vi "Main.vi"(11 "Module Admin":refnum<class "Delacor_lib_QMH_Module Admin.lvclass">) -> ()   [LabVIEW 2024, in "ProductControl.lvlib"]
doc: "This template is based off of the Queued Message Handler design pattern and the Queued Message Handler project template that ships with LabVIEW.\n\nThe main difference is that the queue is private to this module and communication between modules is performed via Broadcast and Request events.\n\nRequest events are wrapped in public API methods and are handled in the Event Handling Loop (EHL) of this VI. Any module can register for Broadcast events sent by this module. The EHL generates messages based on user interface actions.\n\nThe Message Handling Loop (MHL) processes messages generated by the EHL, or by other messages. The messages are string values, so new messages can be added easily to the Message Cases case structure in the MHL. Each message cluster can also provide an optional value for Message Data, which is a variant that can be converted to whatever message-specific data is required.\n_____\nBased on DQMH Dev Tools: Project Template 7.1.0.1503."
uses:
  ProductControl.lvlib
  <vilib>/Delacor/Delacor QMH/Libraries/Module Admin_class/Delacor_lib_QMH_Module Admin.lvclass
  Module Data--cluster.ctl
  <vilib>/Utility/miscctls.llb/LVFontTypeDef.ctl
  Stop Argument--cluster.ctl
  <vilib>/Delacor/Delacor QMH/Libraries/Message Queue_class/Delacor_lib_QMH_Message Queue.lvclass/Delacor_lib_QMH_Message Queue.ctl
  <vilib>/Delacor/Delacor QMH/Libraries/Module Admin_class/Delacor_lib_QMH_Module Admin.lvclass/Delacor_lib_QMH_Module Admin.ctl
  Draw FP in Subpanel Argument--cluster.ctl
  Remove From Subpanel Argument--cluster.ctl
  <vilib>/Delacor/Delacor QMH/Libraries/Message Queue_class/Delacor_lib_QMH_Enqueue Message (Single).vi
  <vilib>/Delacor/Delacor QMH/Libraries/Module Admin_class/Delacor_lib_QMH_Get External Launch.vi
  <vilib>/Delacor/Delacor QMH/Libraries/Message Queue_class/Delacor_lib_QMH_Message Queue.lvclass
  <vilib>/PantherLAB/Message Module/Libraries/Message/PantherLAB_lib_Message.lvlib
panel:
  in  "Productos":i32(listbox)
  out "error out":errorcluster
  out "Status":string
  in  "Comprar":bool
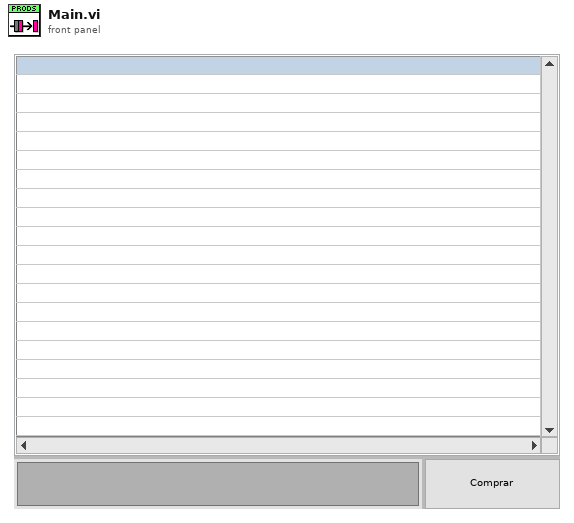
[diagram p1: front panel]
types:
  T1 = typedef "ProductControl.lvlib/Request Events--cluster.ctl" = cluster{"Stop Module":refnum<user-event>, "Show Panel":refnum<user-event>, "Hide Panel":refnum<user-event>, "Get Module Execution Status":refnum<user-event>, "Show Diagram":refnum<user-event>, "Draw FP in Subpanel":refnum<user-event>, "Remove From Subpanel":refnum<user-event>}
  T2 = typedef "PantherLAB_lib_Message.lvlib/Broadcast Events--cluster.ctl" = cluster{"Module Did Init":refnum<user-event>, "Status Updated":refnum<user-event>, "Error Reported":refnum<user-event>, "Module Did Stop":refnum<user-event>, "Update Module Execution Status":refnum<user-event>}
  T3 = typedef "ProductControl.lvlib/Module Data--cluster.ctl" = cluster{"Status":string, "Sub Panel":refnum<vi>}
  T4 = typedef "LVFontTypeDef.ctl" = cluster{"Font Name":string, "Size":u16, "Bold":bool, "Italic":bool, "Underline":bool, "Strikeout":bool, "Color":u32}
  T5 = enum32{"invalid lock state", "Not Locked", "Locked (No Password)", "Password-protected"}
  T6 = typedef "ProductControl.lvlib/Stop Argument--cluster.ctl" = cluster{"Origin":string, "Exit via Stop Module Req?":bool, "Wait for Module to stop?":bool}
  T7 = typedef "ProductControl.lvlib/Draw FP in Subpanel Argument--cluster.ctl" = cluster{"Sub Panel":refnum<vi>}
  T8 = typedef "ProductControl.lvlib/Remove From Subpanel Argument--cluster.ctl" = cluster{"Boolean":bool}
  T9 = enum32{"Invalid", "Standard", "Closed", "Hidden", "Minimized", "Maximized"}
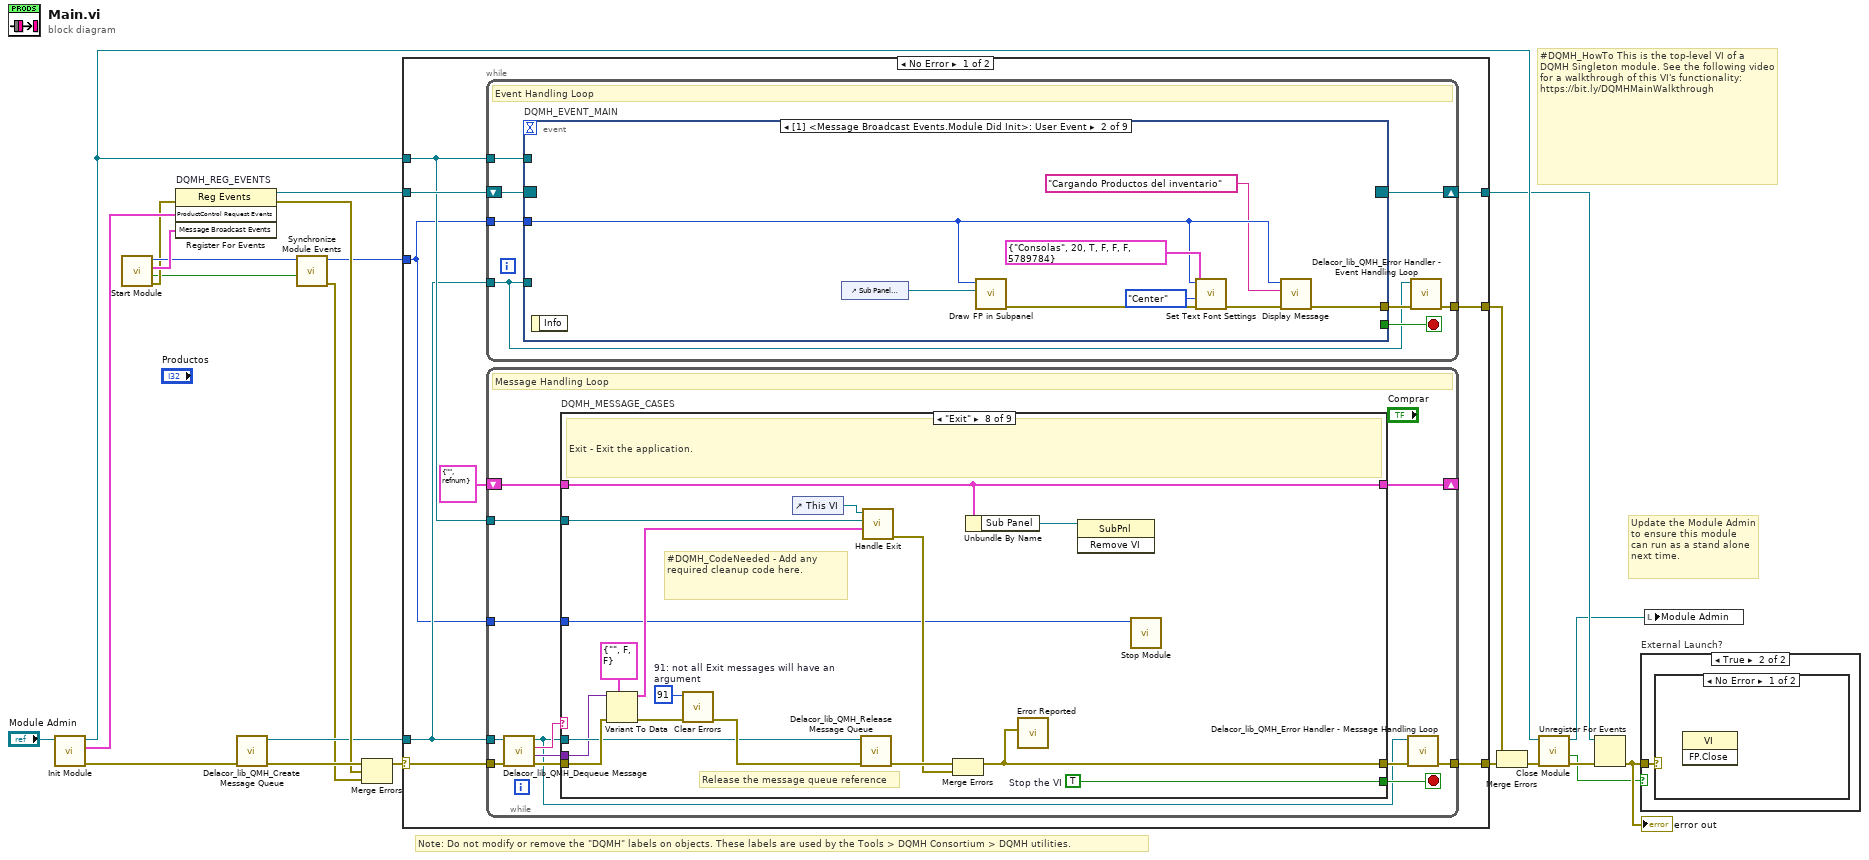
[diagram p0: block diagram]
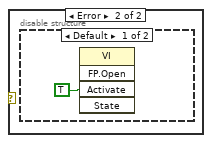
[diagram p3: hidden frame]
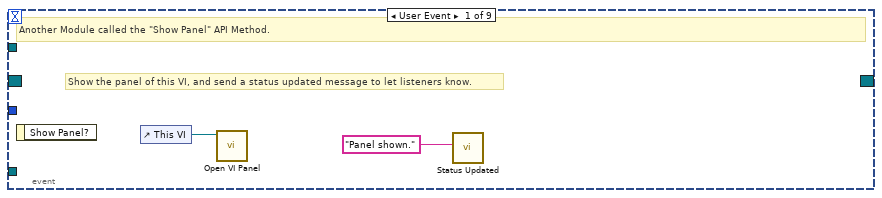
[diagram p5: hidden frame]
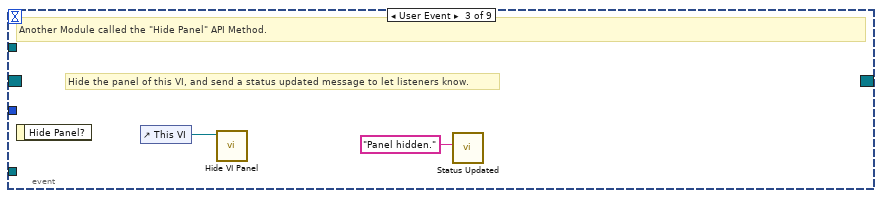
[diagram p6: hidden frame]
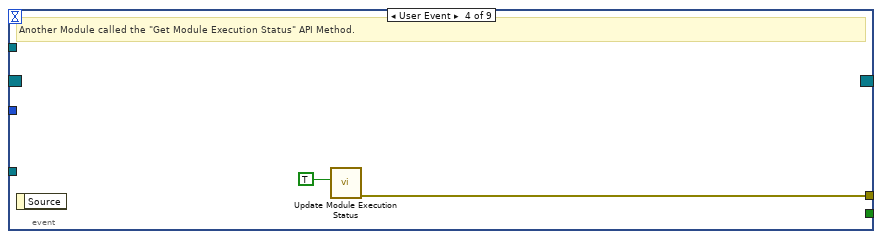
[diagram p7: hidden frame]
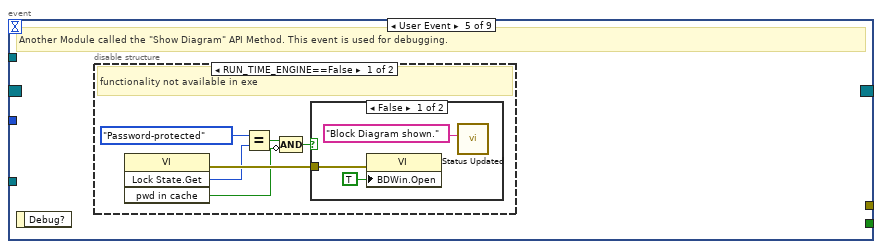
[diagram p8: hidden frame]
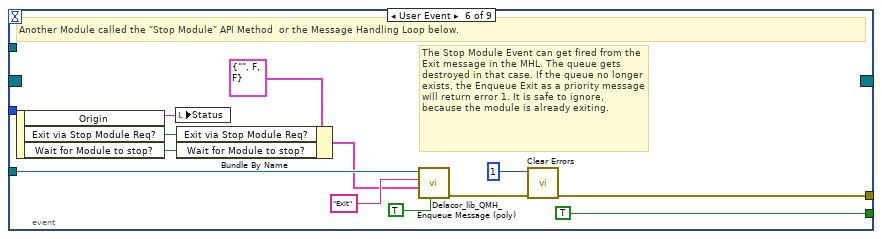
[diagram p11: hidden frame]
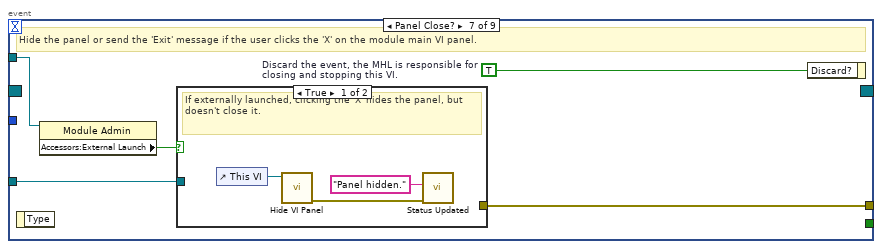
[diagram p12: hidden frame]
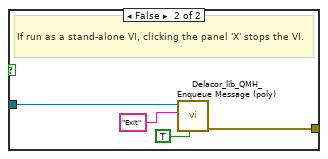
[diagram p13: hidden frame]
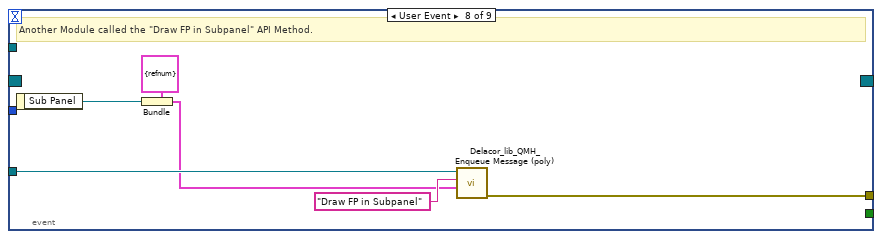
[diagram p14: hidden frame]
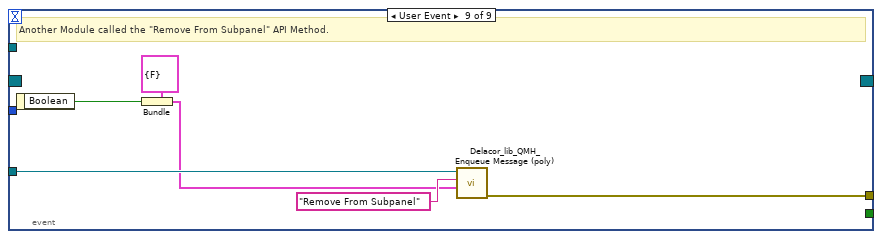
[diagram p15: hidden frame]
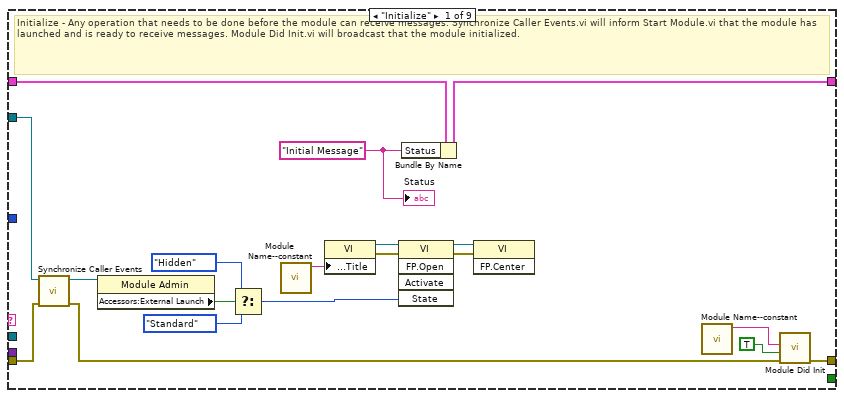
[diagram p16: hidden frame]
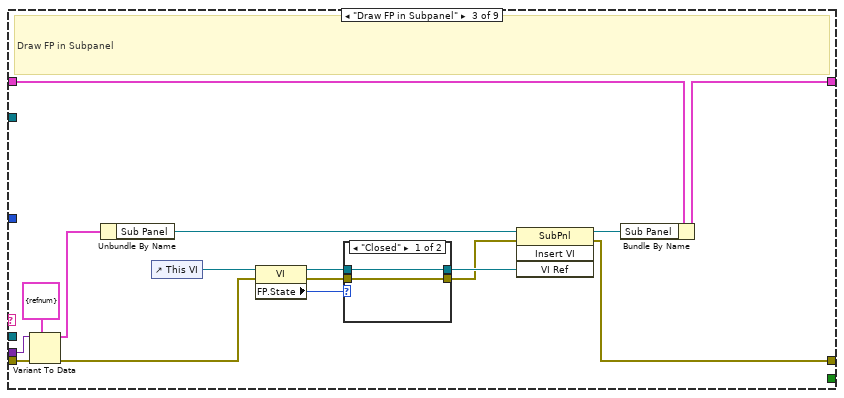
[diagram p18: hidden frame]
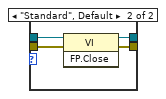
[diagram p19: hidden frame]
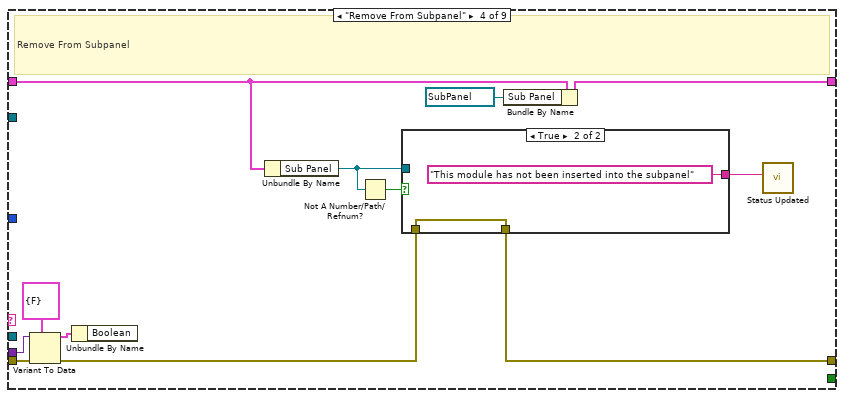
[diagram p20: hidden frame]
diagram:
  # "#DQMH_HowTo This is the top-level VI of a DQMH Singleton module. See the following video for a walkthrough of this VI's functionality: https://bit.ly/DQMHMainWalkthrough"
  # "Note: Do not modify or remove the \"DQMH\" labels on objects. These labels are used by the Tools > DQMH Consortium > DQMH utilities."
  # "Update the Module Admin to ensure this module can run as a stand alone next time."
  n1 = call "Init Module.vi"("Singleton Module Admin in"="Module Admin") -> ("error out"=w22:errorcluster, "ProductControl Request Events"=w11:T1, "Singleton Module Admin out"=w14:refnum<class "Delacor_lib_QMH_Module Admin.lvclass">)  [unwired: 8 in]
  n2 = call <vilib>:"Start Module.vi"() -> ("error out"=w4:errorcluster, "Wait for Event Sync?"=w3:bool, "Message Broadcast Events"=w6:T2, "Module ID"=w5:i32)  [unwired: 7 in, 1 out]
  n3 = register-events "DQMH_REG_EVENTS"(error in=w4, w11, w6) -> (reference out=w12:refnum<event-registration>, error out=w15:errorcluster)  [unwired: 1 in]
  n4 = call <vilib>:"Delacor_lib_QMH_Create Message Queue.vi"("error in"=w22) -> ("error out"=w17:errorcluster, "Message Queue"=w10:refnum<class "Delacor_lib_QMH_Message Queue.lvclass">)  [unwired: 9 in]
  n5 = call <vilib>:"Synchronize Module Events.vi"("Wait for Event Sync?"=w3, "Module ID in"=w5) -> ("error out"=w1:errorcluster, "Module ID out"=w2:i32)  [unwired: 8 in]
  n6 = Merge Errors(w17, w15, w1) -> (w16:errorcluster)
  n7 = case shown="No Error" w16 {
    selector: w16 -> [w30 w231]
    tunnel: [w32 w230] -> w23
    tunnel: [w29 w229] -> w13
    tunnel: w12 -> [w27 w229]
    tunnel: w10 -> [w25 w225]
    tunnel: [w31 _] -> w20
    tunnel: w14 -> [w26 w226]
    tunnel: w2 -> [w24 w224]
    frame No Error {
      n8 = while {
        tunnel: w25 -> [w34]
        shift-right: [w37] -> w29
        shift-left: w27 -> [w38]
        tunnel: [w39] -> w31
        tunnel: w26 -> [w35]
        tunnel: w24 -> [w33]
        stop <- w36 stop-if-true
        # "Event Handling Loop"
        n9 = event "DQMH_EVENT_MAIN" shown="[1] <Message Broadcast Events.Module Did Init>: User Event" {
          selector: w38 -> [_ _ _ _ _ _ _ _ _]
          dyn-events: [_ _ _ _ _ _ _ _ _] -> w37
          timeout: _ -> [_ _ _ _ _ _ _ _ _]
          tunnel: [_ _ _ _ _ TRUE ("Discard?") _ _ _] -> w36
          tunnel: w34 -> [_ _ _ _ _ w71 w78 w93 w99]
          tunnel: [_ w45 _ w54 _ w74 w80 w88 w94] -> w40
          tunnel: w35 -> [_ _ _ _ _ _ w77 _ _]
          tunnel: w33 -> [_ w44 _ _ _ _ _ _ _]
          event User Event {
            # "Show the panel of this VI, and send a status updated message to let listeners know."
            # "Another Module called the \"Show Panel\" API Method."
            n10 = event-data() -> ()  [unwired: 1 in, 1 out]
            n11 = control-ref of="This VI"() -> (w42:refnum<vi>)
            n12 = call "Open VI Panel.vi"("VI"=w42) -> ()  [unwired: 10 in, 1 out]
            n13 = call "Status Updated.vi"("Status"="Panel shown." ("format string")) -> ()  [unwired: 10 in, 1 out]
          }
          event User Event {
            n14 = event-data() -> ()  [unwired: 1 in, 1 out]
            n15 = control-ref of="Sub Panel Mensajes"() -> (w50:refnum<vi>)
            n16 = call <vilib>:"Draw FP in Subpanel.vi"("Sub Panel"=w50, "Module ID"=w44) -> ("error out"=w49:errorcluster)  [unwired: 9 in]
            n17 = call <vilib>:"Set Text Font Settings.vi"("error in"=w49, "Text.Justification"=enum16{"Left", "Center", "Right"}."Center", "Font"=T4 {"Font Name"="Consolas", "Size"=20, "Bold"=TRUE, "Italic"=FALSE, "Underline"=FALSE, "Strikeout"=FALSE, "Color"=5789784}, "Module ID"=w44) -> ("error out"=w46:errorcluster)  [unwired: 7 in]
            n18 = call <vilib>:"Display Message.vi"("error in"=w46, "Message"="Cargando Productos del inventario", "Module ID"=w44) -> ("error out"=w45:errorcluster)  [unwired: 8 in]
          }
          event User Event {
            # "Hide the panel of this VI, and send a status updated message to let listeners know."
            # "Another Module called the \"Hide Panel\" API Method."
            n19 = event-data() -> ()  [unwired: 1 in, 1 out]
            n20 = control-ref of="This VI"() -> (w52:refnum<vi>)
            n21 = call "Hide VI Panel.vi"("VI"=w52) -> ()  [unwired: 10 in, 1 out]
            n22 = call "Status Updated.vi"("Status"="Panel hidden." ("format string")) -> ()  [unwired: 10 in, 1 out]
          }
          event User Event {
            # "Another Module called the \"Get Module Execution Status\" API Method."
            n23 = event-data() -> ()  [unwired: 1 in, 1 out]
            n24 = call "Update Module Execution Status.vi"("Running?"=TRUE) -> ("error out"=w54:errorcluster)  [unwired: 10 in]
          }
          event User Event {
            # "Another Module called the \"Show Diagram\" API Method. This event is used for debugging."
            n25 = event-data() -> ()  [unwired: 1 in, 1 out]
            n26 = disable-structure shown="RUN_TIME_ENGINE==False" {
              frame condition #0 (active) {
                # "functionality not available in exe"
                n27 = invoke on="Invoke Node" class="VI" method="Lock State.Get"() -> (error out=w60:errorcluster, "Get Lock State"=w59:T5, "pwd in cache"=w56:bool)  [unwired: 4 in, 1 out]
                n28 = Equal?(x=T5."Password-protected", y=w59) -> (x = y?=w57:bool)
                n29 = Compound Arithmetic op=AND(w57, invert w56) -> (w55:bool)
                n30 = case shown="False" w55 {
                  tunnel: w60 -> [w63 _]
                  frame False {
                    n31 = property on="Property Node" class="VI"(error in=w63, "BDWin.Open"=TRUE ("Block Diagram Window:Open")) -> ()  [unwired: 1 in, 2 out]
                    n32 = call "Status Updated.vi"("Status"="Block Diagram shown." ("format string")) -> ()  [unwired: 10 in, 1 out]
                  }
                  frame True {
                    # "Password-protected VI, and the password is not in the cache. Do not show the diagram."
                  }
                }
              }
              frame condition #1 {
              }
            }
          }
          event User Event {
            # "The Stop Module Event can get fired from the Exit message in the MHL. The queue gets destroyed in that case. If the queue no longer exists, the Enqueue Exit as a priority message will return error 1. It is safe to ignore, because the module is already exiting."
            # "Another Module called the \"Stop Module\" API Method  or the Message Handling Loop below."
            n33 = event-data() -> ("Origin"=w70:string, "Exit via Stop Module Req?"=w66:bool, "Wait for Module to stop?"=w65:bool)  [unwired: 1 in]
            n34 = local write "Status"(w70) -> ()
            n35 = Bundle By Name(cluster=T6 {"Origin"="", "Exit via Stop Module Req?"=FALSE, "Wait for Module to stop?"=FALSE} ("Stop Argument"), "Exit via Stop Module Req?"=w66, "Wait for Module to stop?"=w65) -> (w64:T6)
            n36 = call-poly <vilib>:"Delacor_lib_QMH_Enqueue Message (poly).vi"("Priority Message? (F)"=TRUE, "Message Data"=w64, "Message"="Exit", "Message Queue in"=w71) -> ("error out"=w75:errorcluster)  [unwired: 6 in, 1 out]
            n37 = call <vilib>:"Clear Errors.vi"("error in (no error)"=w75, "specific error code to clear (0: all)"=1) -> ("error out"=w74:errorcluster)  [unwired: 4 in, 1 out]
          }
          event Panel Close? {
            w79 = TRUE  # Discard the event, the MHL is responsible for closing and stopping this VI.
            # "Hide the panel or send the 'Exit' message if the user clicks the 'X' on the module main VI panel."
            n38 = event-data() -> ()  [unwired: 1 in, 1 out]
            n39 = property on="Property Node" class="Module Admin"(reference=w77) -> ("Accessors:External Launch"=w76:bool)  [unwired: 1 in, 2 out]
            n40 = case shown="True" w76 {
              tunnel: w78 -> [_ w86]
              tunnel: [_ w87] -> w80
              frame True {
                # "If externally launched, clicking the 'X' hides the panel, but doesn't close it."
                n41 = control-ref of="This VI"() -> (w83:refnum<vi>)
                n42 = call "Hide VI Panel.vi"("VI"=w83) -> ("error out"=w81:errorcluster)  [unwired: 10 in]
                n43 = call "Status Updated.vi"("error in"=w81, "Status"="Panel hidden." ("format string")) -> ()  [unwired: 9 in, 1 out]
              }
              frame False {
                # "If run as a stand-alone VI, clicking the panel 'X' stops the VI."
                n44 = call-poly <vilib>:"Delacor_lib_QMH_Enqueue Message (poly).vi"("Priority Message? (F)"=TRUE, "Message"="Exit", "Message Queue in"=w86) -> ("error out"=w87:errorcluster)  [unwired: 7 in, 1 out]
              }
            }
            n45 = event-data ("Event Filter Node")("Discard?"=w79) -> ()  [unwired: 1 in, 1 out]
          }
          event User Event {
            # "Another Module called the \"Draw FP in Subpanel\" API Method."
            n46 = event-data() -> ("Sub Panel"=w89:refnum<vi>)  [unwired: 1 in]
            n47 = Bundle(cluster=T7 {"Sub Panel"=refnum} ("Draw FP in Subpanel Argument"), "Sub Panel"=w89) -> (w90:T7)
            n48 = call-poly <vilib>:"Delacor_lib_QMH_Enqueue Message (poly).vi"("Message Data"=w90, "Message"="Draw FP in Subpanel", "Message Queue in"=w93) -> ("error out"=w88:errorcluster)  [unwired: 7 in, 1 out]
          }
          event User Event {
            # "Another Module called the \"Remove From Subpanel\" API Method."
            n49 = event-data() -> ("Boolean"=w95:bool)  [unwired: 1 in]
            n50 = Bundle(cluster=T8 {"Boolean"=FALSE} ("Remove From Subpanel Argument"), "Boolean"=w95) -> (w96:T8)
            n51 = call-poly <vilib>:"Delacor_lib_QMH_Enqueue Message (poly).vi"("Message Data"=w96, "Message"="Remove From Subpanel", "Message Queue in"=w99) -> ("error out"=w94:errorcluster)  [unwired: 7 in, 1 out]
          }
        }
        n52 = call-dynamic "Delacor_lib_QMH_Error Handler - Event Handling Loop.vi"("error in"=w40, "Message Queue in"=w34) -> ("dup error in"=w39:errorcluster)  [unwired: 8 in, 1 out]
      }
      n53 = while {
        tunnel: w25 -> [w101]
        shift-right: [w109] -> _
        shift-left: T3 {"Status"="", "Sub Panel"=refnum} ("Data Cluster") -> [w110]
        tunnel: w30 -> [w112]
        tunnel: [w104] -> w32
        tunnel: w26 -> [w105]
        tunnel: w24 -> [w100]
        stop <- w108 stop-if-true
        # "Message Handling Loop"
        n54 = call-dynamic "Delacor_lib_QMH_Dequeue Message.vi"("error in"=w112, "Message Queue in"=w101) -> ("error out"=w111:errorcluster, "Message Data"=w106:variant, "Message"=w107:string, "Message Queue out"=w102:refnum<class "Delacor_lib_QMH_Message Queue.lvclass">)  [unwired: 6 in]
        n55 = case "DQMH_MESSAGE_CASES" shown="\"Exit\"" w107 {
          selector: w107 -> [_ _ _ _ _ _ _ _ w218]
          tunnel: w102 -> [_ _ _ _ _ _ w182 w206 _]
          tunnel: w111 -> [w129 w133 w149 w167 w176 w178 w189 w212 w221]
          tunnel: [w127 w133 w141 w161 w175 w178 w185 w207 w222] -> w103
          tunnel: w110 -> [w118 w132 w148 w163 w174 w177 w184 w198 w219]
          tunnel: [w117 w132 w144 w158 w174 w177 w184 w198 w219] -> w109
          tunnel: [_ _ _ _ _ _ _ w205 _] -> w108
          tunnel: w106 -> [_ _ w147 w166 _ _ w183 w204 _]
          tunnel: w105 -> [w119 _ _ _ _ _ w181 w199 _]
          tunnel: w100 -> [_ _ _ _ _ _ _ w196 _]
          frame "Initialize" {
            w113 = "Initial Message" ("Initial Message")
            # "Initialize - Any operation that needs to be done before the module can receive messages. Synchronize Caller Events.vi will inform Start Module.vi that the module has launched and is ready to receive messages. Module Did Init.vi will broadcast that the module initialized."
            n56 = call "Synchronize Caller Events.vi"("error in"=w129, "Singleton Module Admin in"=w119) -> ("error out"=w128:errorcluster, "Singleton Module Admin out"=w114:refnum<class "Delacor_lib_QMH_Module Admin.lvclass">)  [unwired: 8 in]
            n57 = property on="Property Node" class="Module Admin"(reference=w114) -> ("Accessors:External Launch"=w123:bool)  [unwired: 1 in, 2 out]
            n58 = Select(t=T9."Hidden" ("State"), s=w123, f=T9."Standard" ("State")) -> (s? t:f=w120:T9)
            n59 = call "Module Name--constant.vi"() -> ("Module Name"=w126:string)  [unwired: 11 in]
            n60 = property on="Property Node" class="VI"("Front Panel.Title"=w126) -> (reference out=w125:refnum<vi>, error out=w131:errorcluster)  [unwired: 2 in]
            n61 = invoke on="Invoke Node" class="VI" method="FP.Open"(reference=w125, error in=w131, "State"=w120) -> (reference out=w124:refnum<vi>, error out=w130:errorcluster)  [unwired: 2 in, 3 out]
            n62 = Bundle By Name(cluster=w118, "Status"=w113) -> (w117:T3)
            n63 = invoke on="Invoke Node" class="VI" method="FP.Center"(reference=w124, error in=w130) -> ()  [unwired: 1 in, 3 out]
            n64 = call "Module Name--constant.vi"() -> ("Module Name"=w115:string)  [unwired: 11 in]
            n65 = call "Module Did Init.vi"("error in"=w128, "Initialized?"=TRUE, "Origin"=w115) -> ("error out"=w127:errorcluster)  [unwired: 8 in]
            "Status" <- w113
          }
          frame "---Module Specific---" {
            # "Separator -- The following cases handle messages specific to this Module."
          }
          frame "Draw FP in Subpanel" {
            # "Draw FP in Subpanel"
            n66 = Variant To Data(error in=w149, type=T7 {"Sub Panel"=refnum} ("Draw FP in Subpanel Argument"), Variant=w147) -> (data=w145:T7, error out=w139:errorcluster)
            n67 = Unbundle By Name(w145) -> ("Sub Panel"=w143:refnum<vi>)
            n68 = control-ref of="This VI"() -> (w136:refnum<vi>)
            n69 = property class="VI"(reference=w136, error in=w139) -> (reference out=w135:refnum<vi>, error out=w137:errorcluster, "FP.State"=w134:T9)
            n70 = case shown="\"Closed\"" w134 {
              tunnel: [w151 w155] -> w140
              tunnel: [w150 w154] -> w138
              tunnel: w137 -> [w150 w153]
              tunnel: w135 -> [w151 w152]
              frame "Closed" {
              }
              frame "Standard", Default {
                n71 = invoke class="VI" method="FP.Close"(reference=w152, error in=w153) -> (reference out=w155:refnum<vi>, error out=w154:errorcluster)  [unwired: 1 in, 1 out]
              }
            }
            n72 = invoke class="SubPnl" method="Insert VI"(reference=w143, error in=w138, "VI Ref"=w140) -> (reference out=w142:refnum<vi>, error out=w141:errorcluster)  [unwired: 1 in, 2 out]
            n73 = Bundle By Name(cluster=w148, "Sub Panel"=w142) -> (w144:T3)
          }
          frame "Remove From Subpanel" {
            # "Remove From Subpanel"
            n74 = Variant To Data(error in=w167, type=T8 {"Boolean"=FALSE} ("Remove From Subpanel Argument"), Variant=w166) -> (data=w164:T8, error out=w162:errorcluster)
            n75 = Unbundle By Name(w164) -> ()  [unwired: 1 out]
            n76 = Unbundle By Name(w163) -> ("Sub Panel"=w160:refnum<vi>)
            n77 = Not A Number/Path/Refnum?(number/path/refnum=w160) -> (NaN/Path/Refnum?=w159:bool)
            n78 = case shown="True" w159 {
              tunnel: w162 -> [w171 w173]
              tunnel: [w170 w173] -> w161
              tunnel: w160 -> [w169 _]
              tunnel: ["Module Removed from Subpanel" "This module has not been inserted into the subpanel"] -> w156
              frame False {
                n79 = invoke class="SubPnl" method="Remove VI"(reference=w169, error in=w171) -> (error out=w170:errorcluster)  [unwired: 1 in, 2 out]
              }
              frame True {
              }
            }
            n80 = Bundle By Name(cluster=w163, "Sub Panel"=refnum<vi> refnum) -> (w158:T3)
            n81 = call "Status Updated.vi"("Status"=w156) -> ()  [unwired: 10 in, 1 out]
          }
          frame "---Copy This Frame---" {
            # "Duplicate this frame when creating new messages.  Change this comment in the duplicated frame to describe this message."
            n82 = Merge Errors(w176) -> (w175:errorcluster)
          }
          frame "---Exit and Error Handling---" {
            # "Separator - The following cases handle errors and exit messages."
          }
          frame "Error" {
            # "#DQMH_CodeRecommended - If the module is running in standalone mode (External Launch = FALSE), this code will pop up an error dialog and call the 'Exit' message if an error occurs. Add more fine-grained error management here."
            # "Error - Check the error message data and respond accordingly. This message is sent by the \"Error Handler\" VIs at the end of each loop in this application."
            n83 = property on="Property Node" class="Module Admin"(reference=w181) -> ("Accessors:External Launch"=w180:bool)  [unwired: 1 in, 2 out]
            n84 = Variant To Data(error in=w189, type=errorcluster {"status"=FALSE, "code"=0, "source"=""} ("error constant"), Variant=w183) -> (data=w179:errorcluster, error out=w187:errorcluster)
            n85 = local write "error out"(w179) -> ()
            n86 = call "Error Reported.vi"("Error"=w179) -> ()  [unwired: 10 in, 1 out]
            n87 = case shown="False" w180 {
              tunnel: [w194 _] -> w186
              tunnel: w182 -> [w192 _]
              tunnel: w179 -> [w193 _]
              frame False {
                n88 = disable-structure shown="Default" {
                  disable-tunnel: w193 -> [w195 _]
                  frame condition #0 (active) {
                    # "If the module is running standalone, then pop up an error dialog and call the \"Exit\" message."
                    n89 = call <vilib>:"Simple Error Handler.vi"("error in (no error)"=w195) -> ()  [unwired: 4 in, 5 out]
                  }
                  frame condition #1 {
                    # "To prevent the Simple Error Handler VI from being loaded (e.g. when deploying to a Real-Time target), add the Conditional Disable Symbol \"DQMH_Disable_SEH\" to your project and set it to TRUE."
                  }
                }
                n90 = call-poly <vilib>:"Delacor_lib_QMH_Enqueue Message (poly).vi"("Priority Message? (F)"=TRUE, "Message"="Exit", "Message Queue in"=w192) -> ("error out"=w194:errorcluster)  [unwired: 7 in, 1 out]
              }
              frame True {
                # "If the module was launched externally, calling the Error Reported broadcast VI is the only action performed by the \"Error\" message. The module's caller can then process the error appropriately."
              }
            }
            n91 = Merge Errors(w187, w186) -> (w185:errorcluster)
          }
          frame "Exit" {
            w203 = 91  # 91: not all Exit messages will have an argument
            w205 = TRUE  # Stop the VI
            # "Release the message queue reference"
            # "#DQMH_CodeNeeded - Add any required cleanup code here."
            # "Exit - Exit the application."
            n92 = Variant To Data(error in=w212, type=T6 {"Origin"="", "Exit via Stop Module Req?"=FALSE, "Wait for Module to stop?"=FALSE} ("Stop Argument"), Variant=w204) -> (data=w201:T6, error out=w209:errorcluster)
            n93 = call <vilib>:"Clear Errors.vi"("error in (no error)"=w209, "specific error code to clear (0: all)"=w203) -> ("error out"=w211:errorcluster)  [unwired: 4 in, 1 out]
            n94 = control-ref of="This VI"() -> (w200:refnum<vi>)
            n95 = call-dynamic "Delacor_lib_QMH_Release Message Queue.vi"("error in"=w211, "Message Queue"=w206) -> ("error out"=w210:errorcluster)  [unwired: 9 in]
            n96 = call "Handle Exit.vi"("Stop Argument"=w201, "Admin in"=w199, "VI reference"=w200) -> ("error out"=w208:errorcluster)  [unwired: 7 in, 1 out]
            n97 = Merge Errors(w210, w208) -> (w207:errorcluster)
            n98 = Unbundle By Name(w198) -> ("Sub Panel"=w197:refnum<vi>)
            n99 = call "Error Reported.vi"("Error"=w207) -> ()  [unwired: 10 in, 1 out]
            n100 = invoke class="SubPnl" method="Remove VI"(reference=w197) -> ()  [unwired: 2 in, 3 out]
            n101 = call <vilib>:"Stop Module.vi"("Module ID"=w196) -> ()  [unwired: 10 in, 1 out]
          }
          frame Default {
            # "'Default' case only runs if there is a message that isn't defined in any of the other cases.  Output a programming error."
            n102 = call "Module Name--constant.vi"() -> ("Module Name"=w217:string)  [unwired: 11 in]
            n103 = Format Into String(format string="The invalid message string \"%s\" was received in the Message Handling Loop for module \"%s\".", w218, w217) -> (resulting string=w213:string)  [unwired: 2 in, 1 out]
            n104 = call <vilib>:"Error Cluster From Error Code.vi"("show call chain? (False)"=TRUE, "error message (\"\")"=w213, "error code (0)"=1) -> ("error out"=w220:errorcluster)  [unwired: 6 in]
            n105 = Merge Errors(w221, w220) -> (w222:errorcluster)
          }
        }
        n106 = call-dynamic "Delacor_lib_QMH_Error Handler - Message Handling Loop.vi"("error in"=w103, "Message Queue in"=w102) -> ("dup error in"=w104:errorcluster)  [unwired: 8 in, 1 out]
      }
    }
    frame Error {
      # "Synchronize Caller Events.vi will inform Start Module.vi that the module has launched and will let the code calling Start Module.vi register for broadcasts and would permit the caller receive the broadcast that an error occurred at launch time."
      n107 = call-dynamic "Delacor_lib_QMH_Release Message Queue.vi"("error in"=w231, "Message Queue"=w225) -> ("error out"=w230:errorcluster)  [unwired: 9 in]
      n108 = call "Synchronize Caller Events.vi"("Singleton Module Admin in"=w226) -> ("error out"=w232:errorcluster)  [unwired: 9 in, 1 out]
      n109 = call "Module Name--constant.vi"() -> ("Module Name"=w228:string)  [unwired: 11 in]
      n110 = Format Into String(format string="An error occurred during initialization. %s is no longer running.", w228) -> (resulting string=w223:string)  [unwired: 2 in, 1 out]
      n111 = Merge Errors(w230, w232) -> (w233:errorcluster)
      n112 = call "Error Reported.vi"("Additional Information"=w223, "Error"=w233) -> ()  [unwired: 9 in, 1 out]
      n113 = call <vilib>:"Stop Module.vi"("Origin"=w223, "Module ID"=w224) -> ()  [unwired: 9 in, 1 out]
    }
  }
  n114 = Merge Errors(w20, w23) -> (w19:errorcluster)
  n115 = call "Close Module.vi"("error in"=w19, "Module Admin in"=w14) -> ("error out"=w21:errorcluster, "External Launch"=w7:bool, "Module Admin out"=w8:refnum<class "Delacor_lib_QMH_Module Admin.lvclass">)  [unwired: 7 in]
  n116 = Unregister For Events(event registration refnum=w13, error in=w21) -> (error out=w18:errorcluster)
  "error out" <- w18
  n117 = case "External Launch?" shown="True" w7 {
    tunnel: w18 -> [_ w234]
    frame False {
    }
    frame True {
      n118 = case shown="No Error" w234 {
        frame No Error {
          n119 = invoke on="Invoke Node" class="VI" method="FP.Close"() -> ()  [unwired: 3 in, 3 out]
        }
        frame Error {
          n120 = disable-structure shown="Default" {
            frame condition #0 (active) {
              n121 = invoke class="VI" method="FP.Open"("Activate"=TRUE ("Activate?")) -> ()  [unwired: 4 in, 5 out]
            }
            frame condition #1 {
              # "Don't show panel on error if running inside a built EXE."
            }
          }
        }
      }
    }
  }
  n122 = local write "Module Admin"(w8) -> ()
